vi "Motor_Write_MotorSpeed.vi"(8 "error in (no error)":errorcluster, 10 "MotorEncSpeed":dbl[](array[numeric]), 11 "MotorControl in":refnum<class "MotorControl.lvclass">) -> (0 "error out":errorcluster, 3 "MotorControl out":refnum<class "MotorControl.lvclass">)   [LabVIEW 2015, in "MotorControl.lvclass"]
uses:
  MotorControl.lvclass
  MotorControl.lvclass/MotorControl.ctl
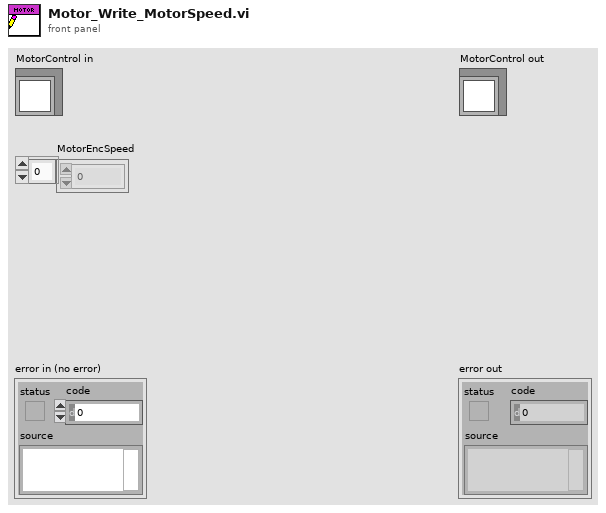
[diagram p1: front panel]
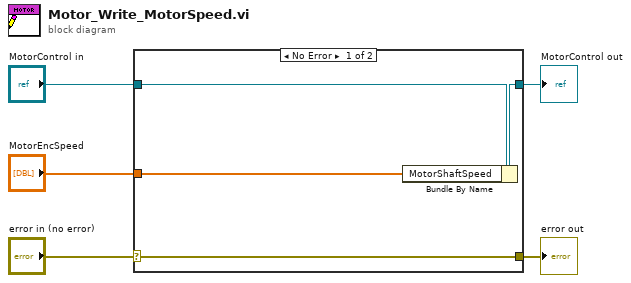
[diagram p0: block diagram]
diagram:
  n1 = case shown="No Error" "error in (no error)" {
    selector: "error in (no error)" -> [w9 w10]
    tunnel: [w9 w10] -> w4
    tunnel: [w7 w11] -> w2
    tunnel: "MotorControl in" -> [w8 w11]
    tunnel: "MotorEncSpeed" -> [w6 _]
    frame No Error {
      n2 = Bundle By Name(cluster=w8, "MotorShaftSpeed"=w6) -> (w7:refnum<class "MotorControl.lvclass">)
    }
    frame Error {
    }
  }
  "error out" <- w4
  "MotorControl out" <- w2
